vi "millisec.vi"() -> ()   [LabVIEW 2017]
uses:
  BERTTA.dll
panel:
  out "increment":i32
  out "time_ms":i32
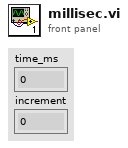
[diagram p1: front panel]
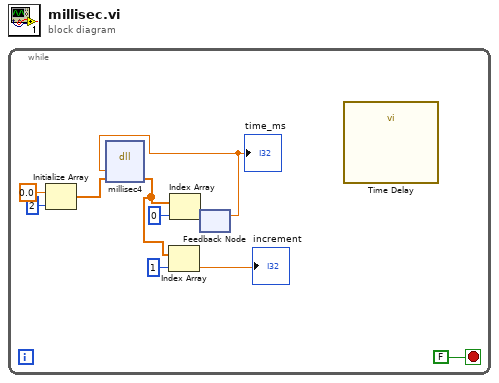
[diagram p0: block diagram]
diagram:
  n1 = while {
    stop <- FALSE stop-if-true
    n2 = Initialize Array(0.0 ("element"), 2 ("dimension size")) -> (w9:dbl[])
    n3 = feedback #1() -> (w1:dbl)  [unwired: 1 in]
    "time_ms" <- w1
    n4 = dll-call lib="C:/Users/p3cn/OneDrive - Kemira Oyj/Documents/GitHub/Bertta/BERTTA/x64/Release/BERTTA.dll" fn="millisec4"("last_time"=w1, "params"=w9) -> ("params"=w4:dbl[])  [unwired: 5 in, 2 out]
    n5 = Index Array(array=w4, index=1) -> (element=→"increment":dbl)
    n6 = Index Array(array=w4, index=0) -> (element=w2:dbl)
    n7 = feedback-in #1(w2) -> ()
    n8 = call "Time Delay"() -> ()  [unwired: 11 in, 1 out]
  }
